vi "Check If Environment Variable Exists.vi"(7 "Target (Process)":T1 items=["Process", "User", "Machine"], 8 "Error In":errorcluster, 11 "Name":string) -> (0 "Error Out":errorcluster, 3 "Exists?":bool)   [LabVIEW 2023, in "SLL Environment Variable.lvlib"]
doc: "Check if the environment variable exists in the target environment."
uses:
  SLL Environment Variable.lvlib
  _Typedef/Target Environment Enum.ctl
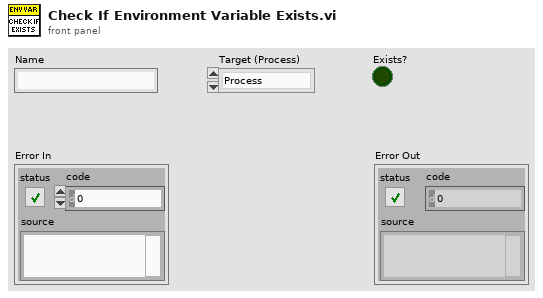
[diagram p1: front panel]
types:
  T1 = typedef "SLL Environment Variable.lvlib/Target Environment Enum.ctl" = i32
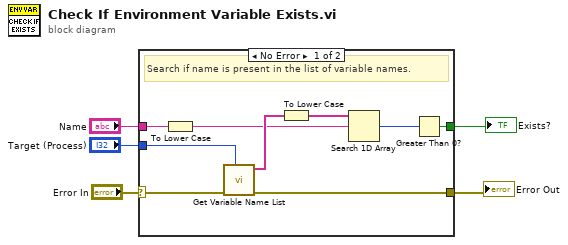
[diagram p0: block diagram]
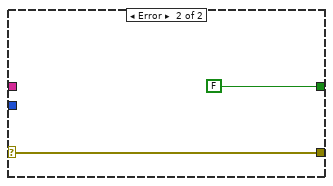
[diagram p2: hidden frame]
diagram:
  n1 = case shown="No Error" "Error In" {
    selector: "Error In" -> [w14 w15]
    tunnel: [w13 w15] -> w4
    tunnel: "Target (Process)" -> [w12 _]
    tunnel: "Name" -> [w10 _]
    tunnel: [w6 FALSE] -> w1
    frame No Error {
      # "Search if name is present in the list of variable names."
      n2 = To Lower Case(string=w10) -> (all lower case string=w9:string)
      n3 = call "Get Variable Name List.vi"("Target (Process)"=w12, "Error In"=w14) -> ("Error Out"=w13:errorcluster, "Names[]"=w11:string[])  [unwired: 8 in]
      n4 = To Lower Case(string=w11) -> (all lower case string=w8:string[])
      n5 = Search 1D Array(1D array=w8, element=w9) -> (index of element=w7:i32)  [unwired: 1 in]
      n6 = Greater Than 0?(x=w7) -> (x > 0?=w6:bool)
    }
    frame Error {
    }
  }
  "Error Out" <- w4
  "Exists?" <- w1
